vi "1K pot drain scheduler.vi"() -> ()   [LabVIEW 2021]
panel:
  in  "Wait voltage":dbl=5.0
  in  "Drain voltage":dbl=10.0
  out "Mode of day":enum16{"day", "night"}(ring)
  out "Time Stamp":timestamp=timestamp(3771605715.57666 s since 1904-01-01) format="%<%I:%M:%S %p>T"
  in  "Daytime end":timestamp=timestamp(-32400 s since 1904-01-01) format="%<%I:%M %p>T"
  in  "Daytime start":timestamp=timestamp(-63000 s since 1904-01-01) format="%<%I:%M %p>T"
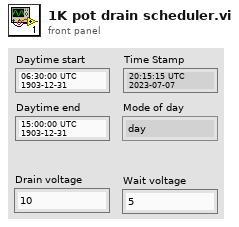
[diagram p1: front panel]
types:
  T1 = enum16{"Set Heater Voltage", "Read Heater Voltage", "Read Heater Current", "Read 1K Pot Temperature", "Read IVC Sorb Temperature", "Read Needle Valve Temperature", "Read Still Pressure", "Read Mixing Chamber Temperature", "Read STM RX Temperature", "Read STM CX Temperature", "Unstall Triton Loop", "Triton Stop", "Triton Stall Status"}
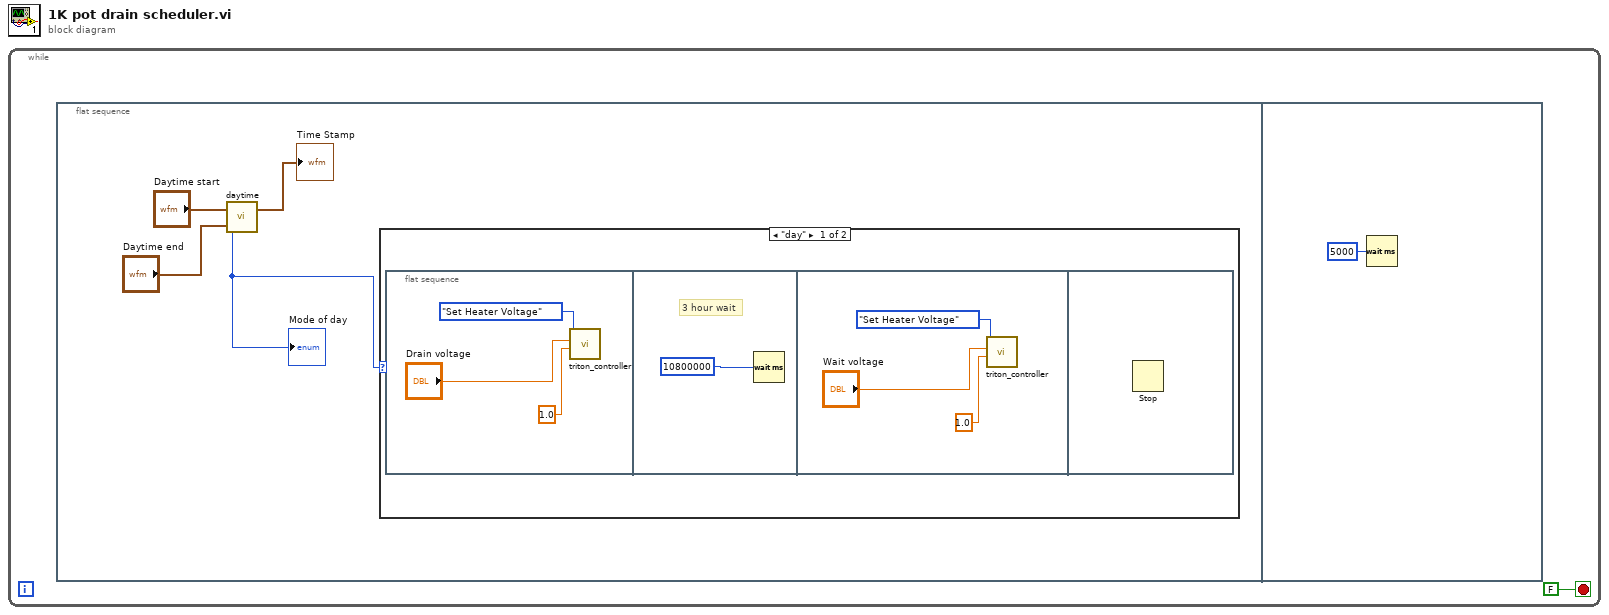
[diagram p0: block diagram]
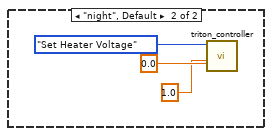
[diagram p2: hidden frame]
diagram:
  n1 = while {
    stop <- FALSE stop-if-true
    n2 = flat-sequence {
      frame #0 {
        n3 = call "daytime.vi"("Daytime end"="Daytime end", "Daytime start"="Daytime start") -> ("Mode of day"=w2:enum16{"day", "night"}, "Time Stamp"=→"Time Stamp":timestamp)
        "Mode of day" <- w2
        n4 = case shown="\"day\"" w2 {
          frame "day" {
            n5 = flat-sequence {
              frame #0 {
                n6 = call "triton_controller.vi"("Increment"=1.0, "Numerical Argument"="Drain voltage", "Command"=T1."Set Heater Voltage") -> ()  [unwired: 8 in, 1 out]
              }
              frame #1 {
                # "3 hour wait"
                n7 = Wait (ms)(milliseconds to wait=u32 10800000) -> ()  [unwired: 1 out]
              }
              frame #2 {
                n8 = call "triton_controller.vi"("Increment"=1.0, "Numerical Argument"="Wait voltage", "Command"=T1."Set Heater Voltage") -> ()  [unwired: 8 in, 1 out]
              }
              frame #3 {
                n9 = Stop() -> ()  [unwired: 1 in]
              }
            }
          }
          frame "night", Default {
            n10 = call "triton_controller.vi"("Increment"=1.0, "Numerical Argument"=0.0, "Command"=T1."Set Heater Voltage") -> ()  [unwired: 8 in, 1 out]
          }
        }
      }
      frame #1 {
        n11 = Wait (ms)(milliseconds to wait=u32 5000) -> ()  [unwired: 1 out]
      }
    }
  }
